vi "UPortal Open URL.vi"(4 "Found":bool, 5 "MagLab User Name":string, 6 "URL":string, 7 "notifier in":refnum<notifier>, 8 "error in (no error)":errorcluster, 9 "User portal URL":string, 10 "Password":string, 11 ".NET Refnum in":refnum<k24>) -> (0 "error out":errorcluster, 3 "time lapsed":u32 format="%.0fms")   [LabVIEW 2020]
uses:
  System.Windows.Forms
panel:
  out "URL":string
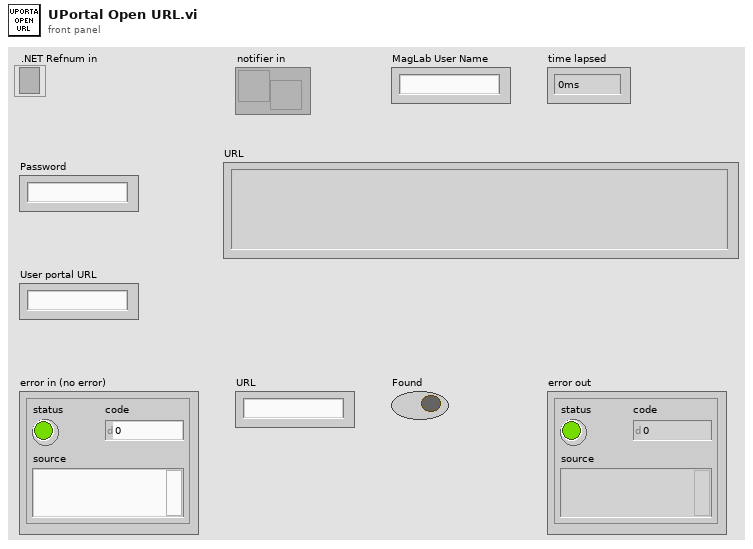
[diagram p1: front panel]
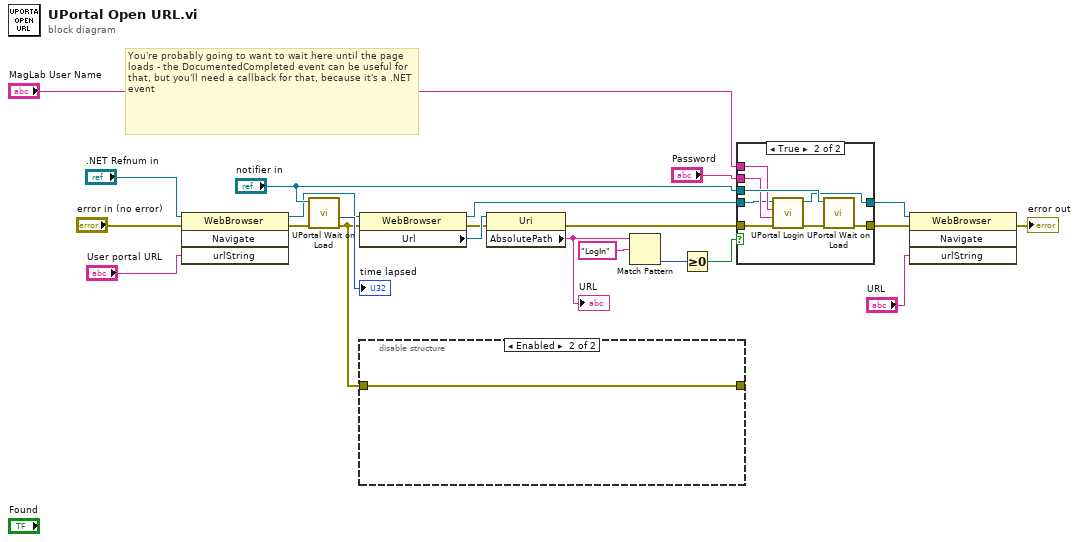
[diagram p0: block diagram]
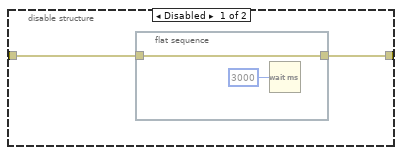
[diagram p3: hidden frame]
diagram:
  # "You're probably going to want to wait here until the page loads - the DocumentedCompleted event can be useful for that, but you'll need a callback for that, because it's a .NET event"
  n1 = invoke class="WebBrowser" method="Navigate"(reference=".NET Refnum in", error in="error in (no error)", "urlString"="User portal URL") -> (reference out=w3:refnum<k24>, error out=w15:errorcluster)  [unwired: 1 in, 2 out]
  n2 = call "UPortal Wait on Load.vi"("error in"=w15, "notifier"="notifier in") -> ("error out"=w10:errorcluster, "time lapsed"=→"time lapsed":u32)  [unwired: 6 in, 2 out]
  n3 = property class="WebBrowser"(reference=w3, error in=w10) -> (reference out=w2:refnum<k24>, error out=w5:errorcluster, "Url"=w9:refnum<k24>)
  n4 = disable-structure shown="Enabled" {
    disable-tunnel: w10 -> [w24 w27]
    disable-tunnel: [w23 w27] -> _
    frame Disabled {
      n5 = flat-sequence {
        tunnel: w24 -> [w25]
        tunnel: [w25] -> w23
        frame #0 {
          n6 = Wait (ms)(milliseconds to wait=u32 3000) -> ()  [unwired: 1 out]
        }
      }
    }
    frame Enabled {
    }
  }
  n7 = property class="Uri"(reference=w9, error in=w5) -> (error out=w4:errorcluster, "AbsolutePath"=w1:string)  [unwired: 1 out]
  "URL" <- w1
  n8 = Match Pattern(string=w1, regular expression="LogIn") -> (offset past match=w7:i32)  [unwired: 1 in, 3 out]
  n9 = Greater Or Equal To 0?(x=w7) -> (x >= 0?=w6:bool)
  n10 = case shown="True" w6 {
    tunnel: "notifier in" -> [_ w37]
    tunnel: [w29 w36] -> w20
    tunnel: [w28 w34] -> w18
    tunnel: "Password" -> [_ w33]
    tunnel: "MagLab User Name" -> [_ w32]
    tunnel: w2 -> [w28 w31]
    tunnel: w4 -> [w29 w30]
    frame False {
    }
    frame True {
      n11 = call "UPortal Login.vi"("error in"=w30, "Password"=w33, "User name"=w32, "Browser reference"=w31) -> ("error out"=w35:errorcluster, "Browser reference out"=w34:refnum<k24>)  [unwired: 6 in]
      n12 = call "UPortal Wait on Load.vi"("error in"=w35, "notifier"=w37) -> ("error out"=w36:errorcluster)  [unwired: 6 in, 3 out]
    }
  }
  n13 = invoke class="WebBrowser" method="Navigate"(reference=w18, error in=w20, "urlString"="URL") -> (error out=→"error out":errorcluster)  [unwired: 1 in, 3 out]
